vi "SD Write Value.vi"   [LabVIEW 2017]
doc: "A polymorphic VI that will write the data to the SmartDashboard entry -- /prefix/name. It adapts to the type wired to it."
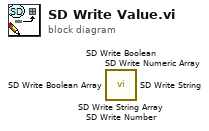
[diagram p0: block diagram]
diagram:
  n1 = call <vilib>:"SD Write String Array.vi"() -> ()  [unwired: 10 in, 2 out]
  n2 = call <vilib>:"SD Write Numeric Array.vi"() -> ()  [unwired: 10 in, 2 out]
  n3 = call <vilib>:"SD Write Boolean Array.vi"() -> ()  [unwired: 10 in, 2 out]
  n4 = call <vilib>:"SD Write String.vi"() -> ()  [unwired: 10 in, 2 out]
  n5 = call <vilib>:"SD Write Number.vi"() -> ()  [unwired: 10 in, 2 out]
  n6 = call <vilib>:"SD Write Boolean.vi"() -> ()  [unwired: 10 in, 2 out]
